vi "读取组属性.vi"(5 "tdms文件输出":refnum<k34>, 7 "组名称":string, 8 "属性名称":string[](array[string]), 10 "属性值":variant[](array[variant]), 11 "错误输入（无错误）":errorcluster) -> (0 "测试数据":T1, 1 "数据类型":string, 3 "错误输出":errorcluster)   [LabVIEW 2021]
uses:
  LabView Lib/Base64/Base64.lvlib
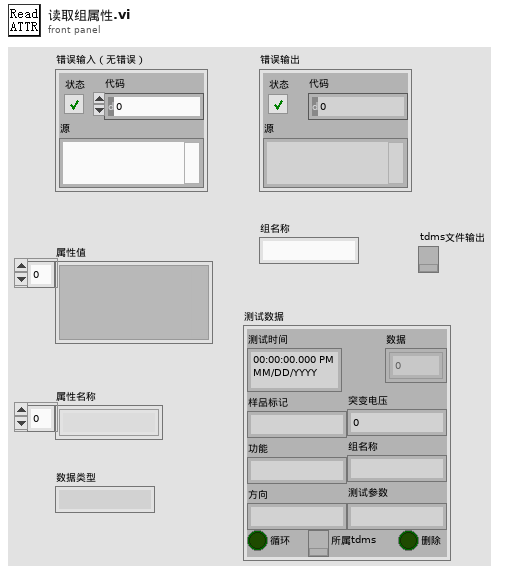
[diagram p1: front panel]
types:
  T1 = typedef "测试数据类型.ctl" = cluster{"测试时间":timestamp, "数据":dbl[][], "功能":string, "方向":string, "循环":bool, "样品标记":string, "突变电压":i32, "所属tdms":refnum<k34>, "组名称":string, "删除":bool, "测试参数":string}
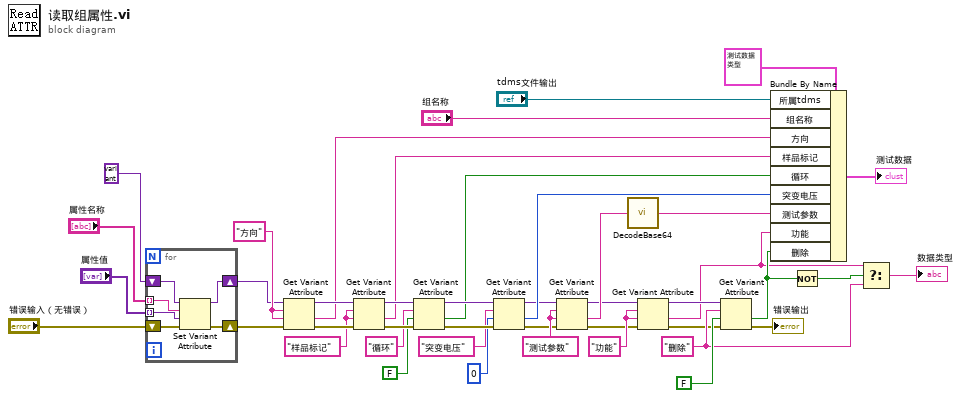
[diagram p0: block diagram]
diagram:
  w42 = "测试参数" ("名称")
  w14 = "删除" ("名称")
  w32 = "样品标记" ("名称")
  w33 = "方向" ("名称")
  w19 = "功能" ("名称")
  n1 = for {
    tunnel: "属性名称" -> [w49] mode=indexing
    tunnel: "属性值" -> [w48] mode=indexing
    shift-right: [w47] -> w5
    shift-left: variant -> [w46]
    shift-right: [w44] -> w4
    shift-left: "错误输入（无错误）" -> [w45]
    n2 = Set Variant Attribute(Variant=w46, name=w49, value=w48, error in=w45) -> (Variant out=w47:variant, error out=w44:errorcluster)  [unwired: 1 out]
  }
  n3 = Get Variant Attribute(Variant=w5, name=w33, default value (empty Variant)=w33, error in=w4) -> (duplicate Variant=w26:variant, value=w20:string, error out=w36:errorcluster)  [unwired: 1 out]
  n4 = Get Variant Attribute(Variant=w26, name=w32, default value (empty Variant)=w32, error in=w36) -> (duplicate Variant=w25:variant, value=w23:string, error out=w37:errorcluster)  [unwired: 1 out]
  n5 = Get Variant Attribute(Variant=w25, name="循环" ("名称"), default value (empty Variant)=FALSE, error in=w37) -> (duplicate Variant=w24:variant, value=w22:bool, error out=w38:errorcluster)  [unwired: 1 out]
  n6 = Get Variant Attribute(Variant=w24, name="突变电压" ("名称"), default value (empty Variant)=0, error in=w38) -> (duplicate Variant=w8:variant, value=w21:i32, error out=w7:errorcluster)  [unwired: 1 out]
  n7 = Get Variant Attribute(Variant=w8, name=w42, default value (empty Variant)=w42, error in=w7) -> (duplicate Variant=w9:variant, value=w43:string, error out=w1:errorcluster)  [unwired: 1 out]
  n8 = call "DecodeBase64.vi"("Base64"=w43) -> ("Data"=w6:string)
  n9 = Get Variant Attribute(Variant=w9, name=w19, default value (empty Variant)=w19, error in=w1) -> (duplicate Variant=w13:variant, value=w10:string, error out=w11:errorcluster)  [unwired: 1 out]
  n10 = Get Variant Attribute(Variant=w13, name=w14, default value (empty Variant)=FALSE, error in=w11) -> (value=w40:bool, error out=→"错误输出":errorcluster)  [unwired: 2 out]
  n11 = Bundle By Name(cluster=T1 {"测试时间"=timestamp(0 s since 1904-01-01), "数据"=[], "功能"="", "方向"="", "循环"=FALSE, "样品标记"="", "突变电压"=0, "所属tdms"=refnum, "组名称"="", "删除"=FALSE, "测试参数"=""} ("测试数据"), "所属tdms"="tdms文件输出", "组名称"="组名称", "方向"=w20, "样品标记"=w23, "循环"=w22, "突变电压"=w21, "测试参数"=w6, "功能"=w10, "删除"=w40) -> (→"测试数据":T1)
  n12 = Not(x=w40) -> (.not. x?=w15:bool)
  n13 = Select(t=w10, s=w15, f=w14) -> (s? t:f=→"数据类型":string)
